vi "CODMn通讯.vi"() -> ()   [LabVIEW 2016, in "斯坦道CODMn.lvlib"]
uses:
  <vilib>/NI/Modbus Library/API/Wrapper/Create TCP Slave.vi
  <vilib>/NI/Modbus Library/API/slave/Modbus Slave.lvclass
  <vilib>/Plasmionique/MB Master/MB_Master/MB_Master.lvclass
  <vilib>/Plasmionique/MB Master/MB Master.lvlib
  <vilib>/Utility/config.llb/NI_LVConfig.lvlib
  <vilib>/NI/Modbus Library/API/Wrapper/API Main.lvlib
panel:
  in  "读取数据":bool
  in  "释放串口":bool
  in  "打开串口":bool
  out "队列中元素数量":i32
  out "元素":cluster{"命令":string}[](array[cluster])
  out "待处理插入数量":i32
  out "读取公式":u16[](array[numeric])
  out "读取参数":u16[](array[numeric])
  out "数据存储":u16[](array[numeric])
  out "温度":bool[](array[boolean])
  out "M输出点":bool[](array[boolean])
  out "ORP、时间":u16[](array[numeric])
  out "测量状态":u16[](array[numeric])
  out "通讯状态":bool
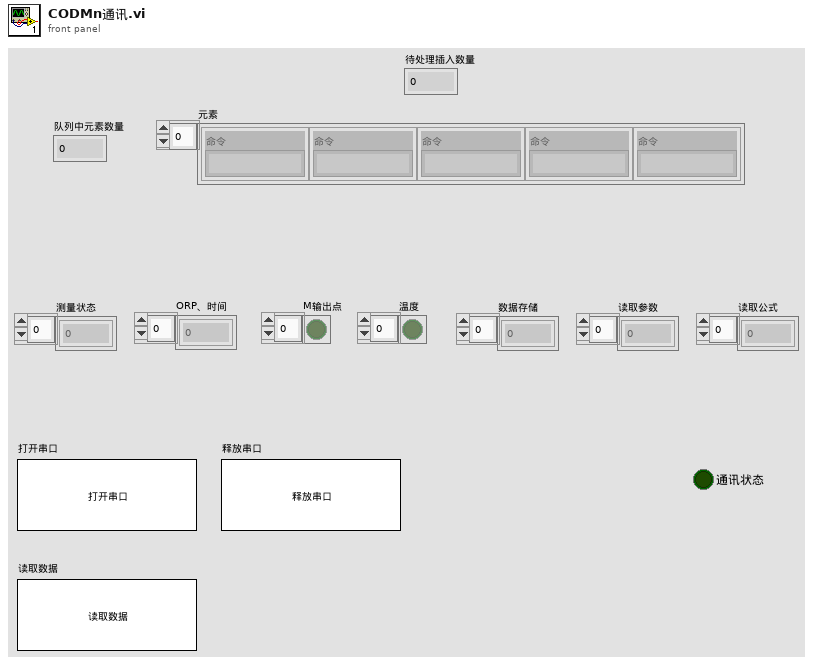
[diagram p1: front panel]
types:
  T1 = cluster{"命令":string, "测量模式":enum16{"水样测量", "标样核查", "零点核查", "跨度核查", "空白测试", "加标回收", "平行样", "校零", "校标"}, "CODMn量程切换":enum32{"H", "L", "AUTO"}}
  T2 = typedef "NI_LVConfig.lvlib/Config Data RefNum.ctl" = refnum<k1>
  T3 = enum16{"空闲", "水样测试", "标样核查", "零点核查", "跨度核查", "空白测试", "平行样测试", "质控样", "空白校准", "标样校准", "加标回收"}
  T4 = enum16{"水样测量", "标样核查", "零点核查", "跨度核查", "空白测试", "加标回收", "平行样", "校零", "校标"}
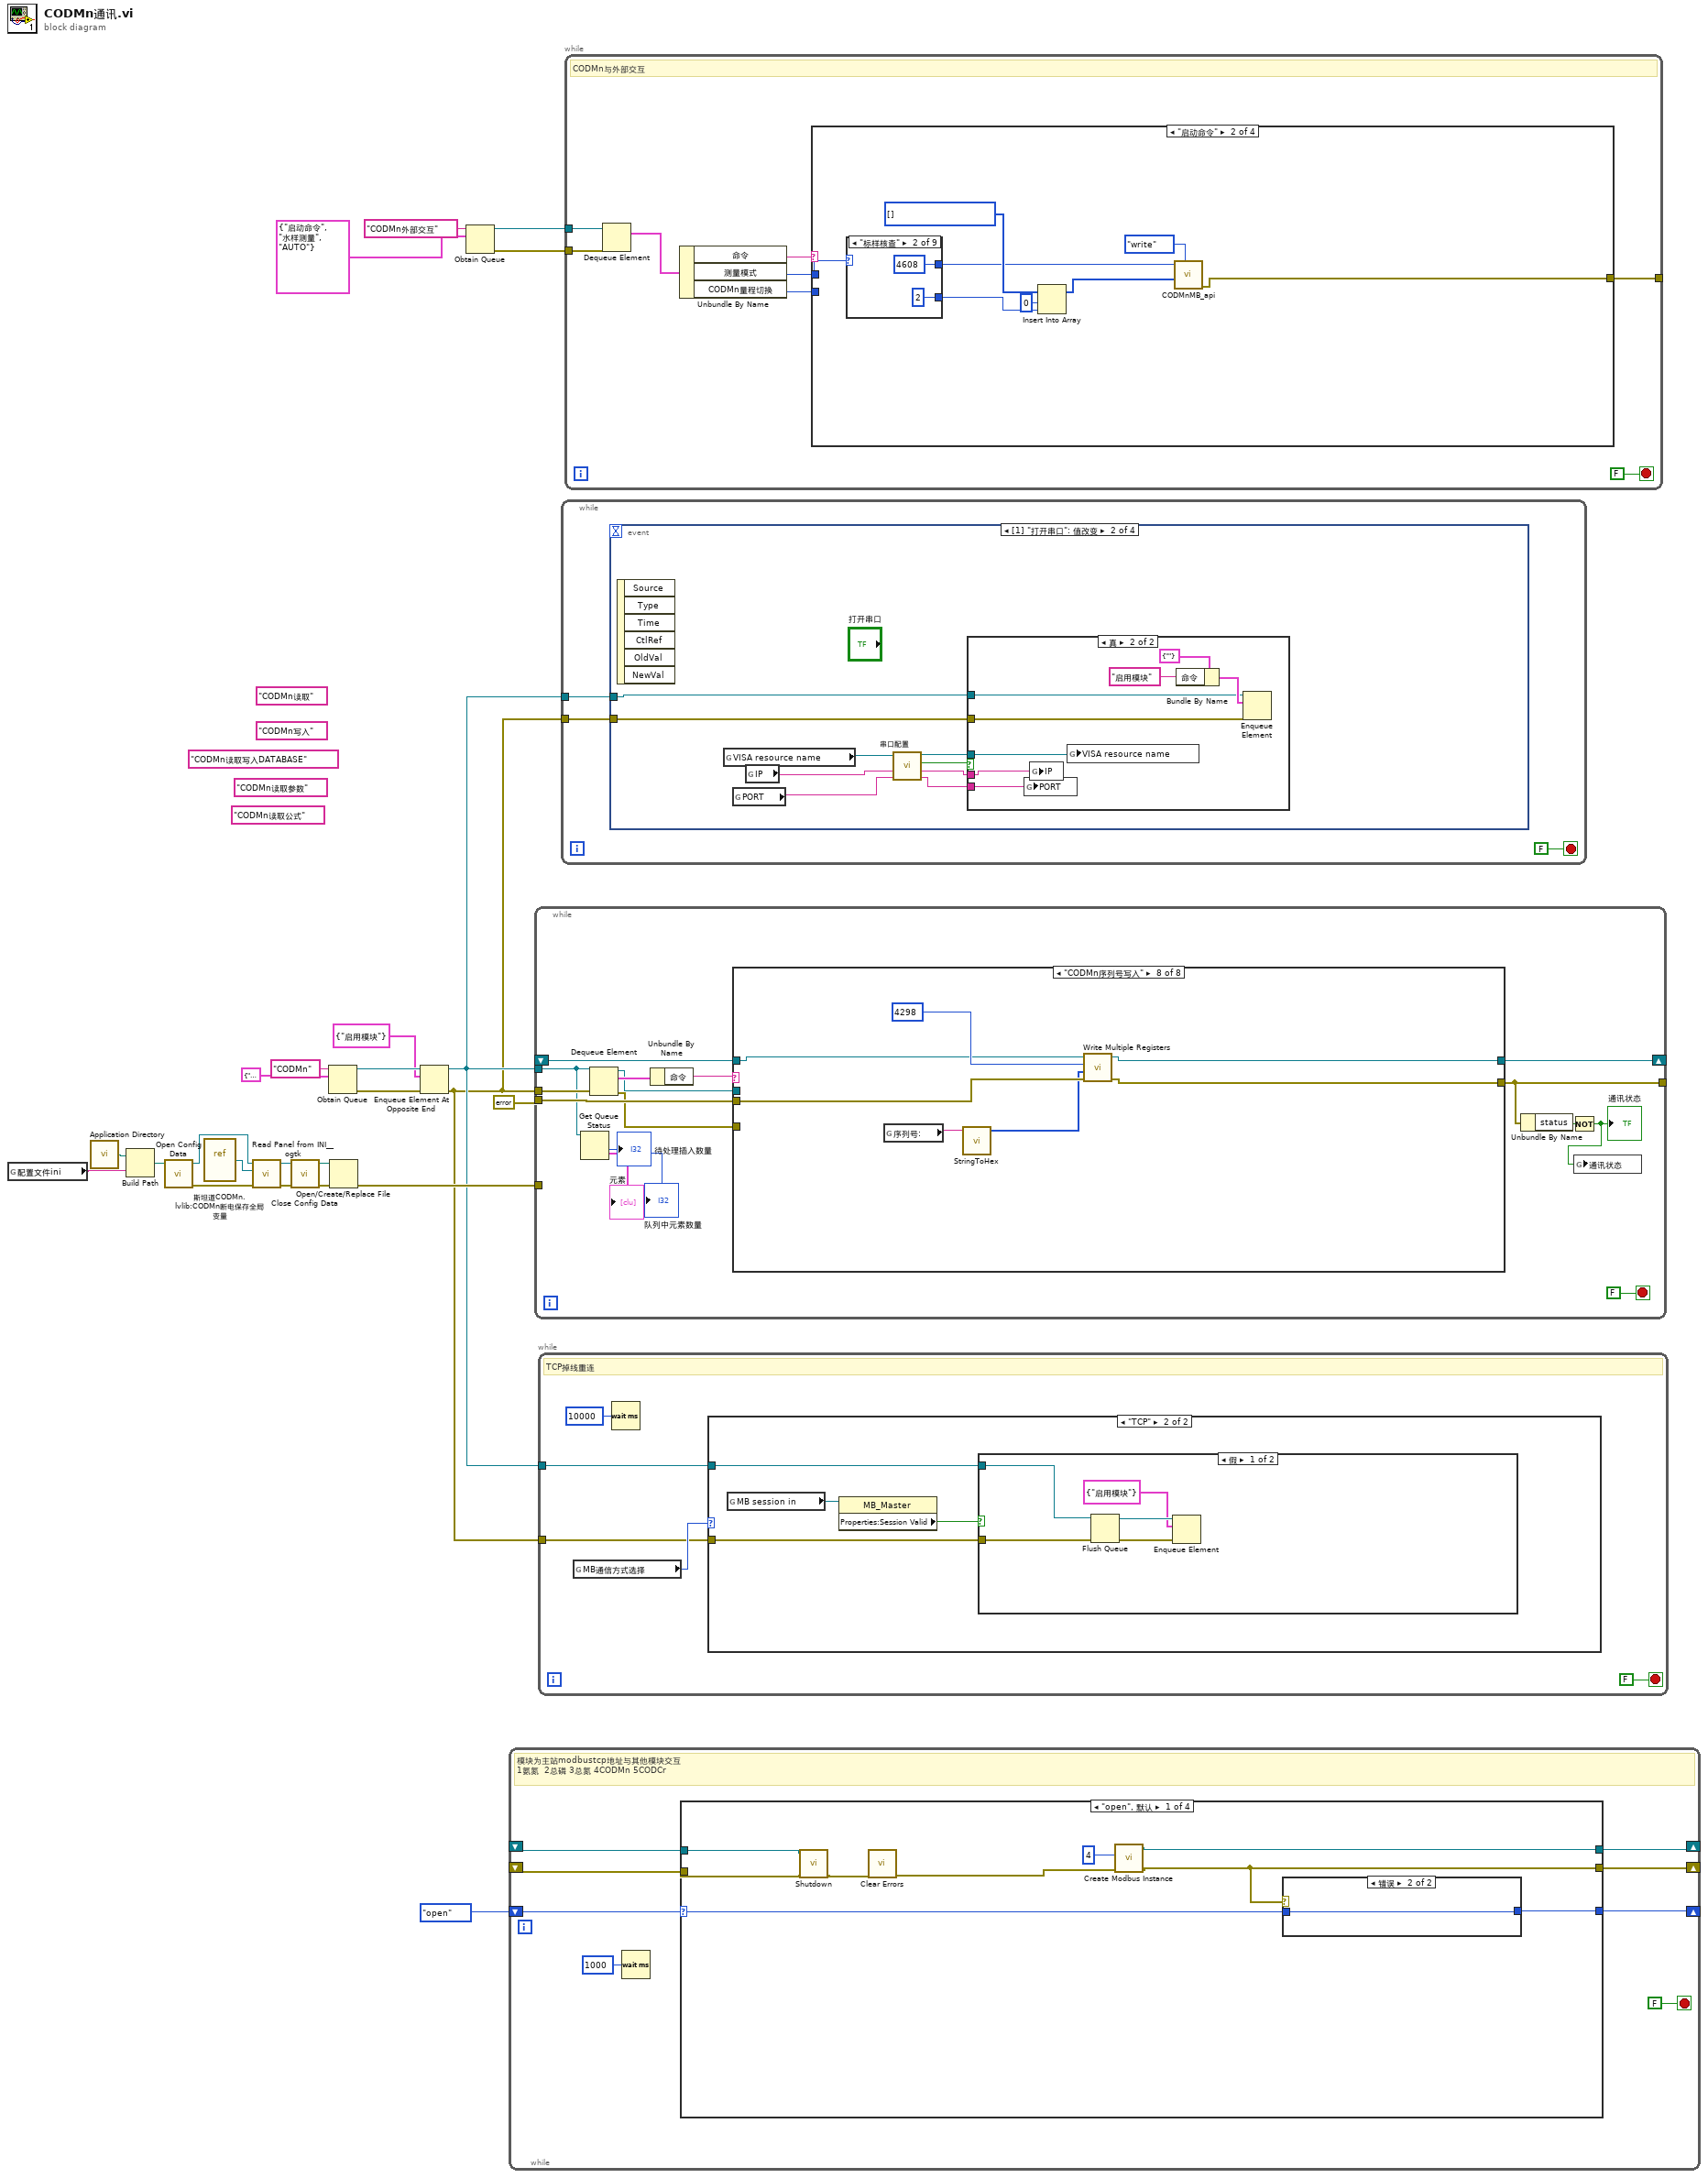
[diagram p0: block diagram]
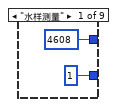
[diagram p3: hidden frame]
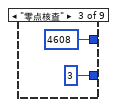
[diagram p4: hidden frame]
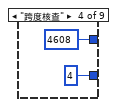
[diagram p5: hidden frame]
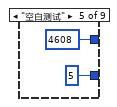
[diagram p6: hidden frame]
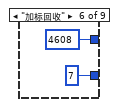
[diagram p7: hidden frame]
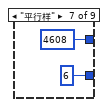
[diagram p8: hidden frame]
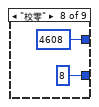
[diagram p9: hidden frame]
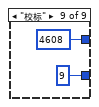
[diagram p10: hidden frame]
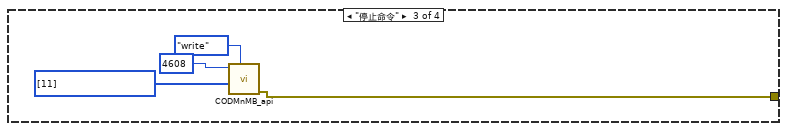
[diagram p11: hidden frame]
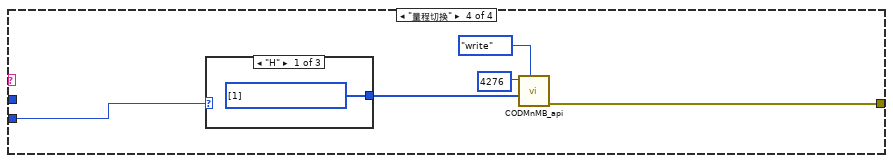
[diagram p12: hidden frame]
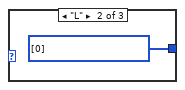
[diagram p13: hidden frame]
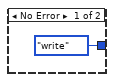
[diagram p17: hidden frame]
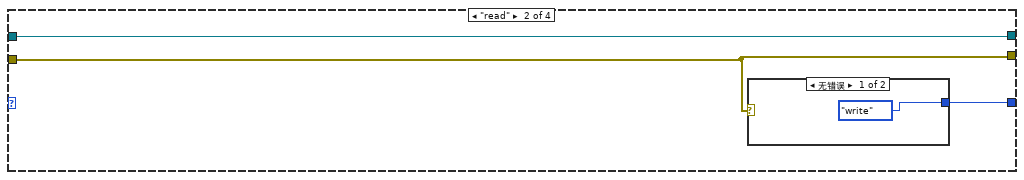
[diagram p18: hidden frame]
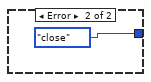
[diagram p19: hidden frame]
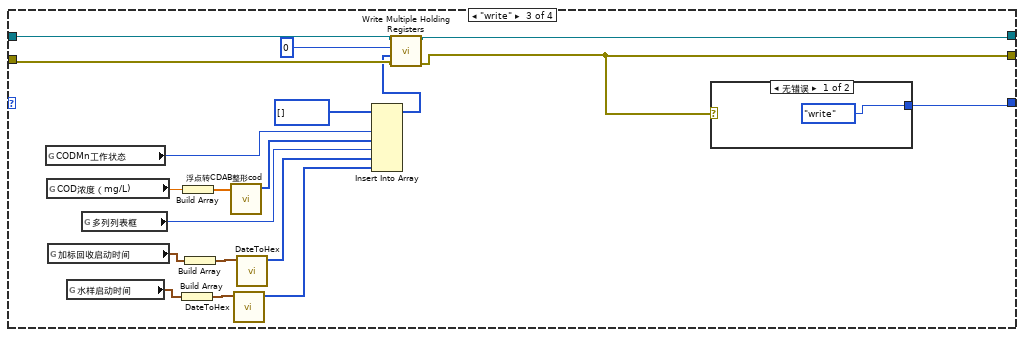
[diagram p20: hidden frame]
diagram:
  (unwired) "CODMn读取公式" ("名称（未命名）")
  (unwired) "CODMn读取写入DATABASE" ("名称（未命名）")
  (unwired) "CODMn读取参数" ("名称（未命名）")
  (unwired) "CODMn读取" ("名称（未命名）")
  (unwired) "CODMn写入" ("名称（未命名）")
  n1 = global read "COD内部交互全局.vi" "配置文件ini"() -> (w5:string)
  n2 = call <vilib>:"Application Directory.vi"() -> ("Application Directory"=w18:path)
  n3 = Build Path(base path=w18, name or relative path=w5) -> (appended path=w17:path)
  n4 = call <vilib>:"Open Config Data.vi"("configuration file path"=w17) -> ("error out"=w13:errorcluster, "refnum"=w16:T2)  [unwired: 8 in, 1 out]
  n5 = vi-ref "斯坦道CODMn.lvlib:CODMn断电保存全局变量.vi"() -> (w15:refnum<vi>)
  n6 = call <userlib>:"Read Panel from INI__ogtk.vi"("error in (no error)"=w13, "VI ref"=w15, "refnum"=w16) -> ("error out"=w12:errorcluster, "refnum out"=w14:T2)  [unwired: 7 in]
  n7 = call <vilib>:"Close Config Data.vi"("error in (no error)"=w12, "refnum"=w14) -> ("error out"=w11:errorcluster, "file path"=w10:path)  [unwired: 8 in]
  n8 = Obtain Queue(name (unnamed)="CODMn" ("名称（未命名）"), element data type=cluster{"命令":string} {"命令"="启用模块"} ("元素")) -> (queue out=w21:refnum<queue>, error out=w20:errorcluster)  [unwired: 3 in, 1 out]
  n9 = Open/Create/Replace File(file path (use dialog)=w10, error in=w11) -> (error out=w9:errorcluster)  [unwired: 4 in, 2 out]
  n10 = Enqueue Element At Opposite End(queue=w21, element=cluster{"命令":string} {"命令"="启用模块"} ("元素"), error in (no error)=w20) -> (queue out=w7:refnum<queue>, error out=w6:errorcluster)  [unwired: 1 in, 1 out]
  n11 = Obtain Queue(name (unnamed)="CODMn外部交互" ("名称（未命名）"), element data type=T1 {"命令"="启动命令", "测量模式"=enum."水样测量", "CODMn量程切换"=enum."AUTO"} ("元素")) -> (queue out=w2:refnum<queue>, error out=w1:errorcluster)  [unwired: 3 in, 1 out]
  n12 = while {
    shift-right: [w30] -> _
    shift-left: _ -> [w32]
    shift-right: [w29] -> _
    shift-left: _ -> [w31]
    shift-right: [w26] -> _
    shift-left: enum16{"open", "read", "write", "close"}."open" -> [w27]
    stop <- FALSE stop-if-true
    # "模块为主站modbustcp地址与其他模块交互\n1氨氮  2总磷 3总氮 4CODMn 5CODCr"
    n13 = Wait (ms)(milliseconds to wait=u32 1000 ("等待时间（毫秒）")) -> ()  [unwired: 1 out]
    n14 = case shown="\"open\", 默认" w27 {
      selector: w27 -> [w41 _ _ _]
      tunnel: w32 -> [w35 w44 w66 w72]
      tunnel: w31 -> [w34 w45 w63 w71]
      tunnel: [w38 w44 w65 w72] -> w30
      tunnel: [w37 w45 w64 w74] -> w29
      tunnel: [w40 w46 w67 enum16{"open", "read", "write", "close"}."open"] -> w26
      frame "open", Default {
        n15 = call-dynamic "Shutdown.vi"("error in"=w34, "Modbus slave in"=w35) -> ("error out"=w33:errorcluster)  [unwired: 9 in]
        n16 = call <vilib>:"Clear Errors.vi"("error in (no error)"=w33) -> ("error out"=w36:errorcluster)  [unwired: 5 in, 1 out]
        n17 = call-poly <vilib>:"Create Modbus Instance.vi"("error in"=w36, "port (502)"=u16 4) -> ("error out"=w37:errorcluster, "TCP slave instance"=w38:refnum<class "Modbus Slave.lvclass">)  [unwired: 8 in]
        n18 = case shown="错误" w37 {
          tunnel: w41 -> [_ w43]
          tunnel: [enum16{"open", "read", "write", "close"}."write" w43] -> w40
          frame No Error {
          }
          frame Error {
          }
        }
      }
      frame "read" {
        n19 = case shown="无错误" w45 {
          tunnel: [enum16{"open", "read", "write", "close"}."write" enum16{"open", "read", "write", "close"}."close"] -> w46
          frame No Error {
          }
          frame Error {
          }
        }
      }
      frame "write" {
        n20 = global read "COD测量模式全局.vi" "CODMn工作状态"() -> (w53:T3)
        n21 = global read "COD浓度全局变量.vi" "COD浓度（mg/L)"() -> (w55:dbl)
        n22 = global read "COD测量模式全局.vi" "加标回收启动时间"() -> (w58:timestamp)
        n23 = global read "COD测量模式全局.vi" "水样启动时间"() -> (w60:timestamp)
        n24 = global read "运行时序全局变量.vi" "多列列表框"() -> (w57:i32)
        n25 = Build Array(w60) -> (w59:timestamp[])
        n26 = Build Array(w55) -> (w54:dbl[])
        n27 = Build Array(w58) -> (w51:timestamp[])
        n28 = call "浮点转CDAB整形cod.vi"("浮点数"=w54) -> ("CDAB整形输出"=w56:u16[])  [unwired: 10 in]
        n29 = call "DateToHex.vi"("DATE"=w59) -> ("数组"=w62:u16[])  [unwired: 10 in]
        n30 = call "DateToHex.vi"("DATE"=w51) -> ("数组"=w61:u16[])  [unwired: 10 in]
        n31 = Insert Into Array(array=u16[] [] ("values"), new element #1=w53, new element #2=w56, new element #3=w57, new element #4=w61, new element #5=w62) -> (w50:u16[])  [unwired: 1 in]
        n32 = call-dynamic "Write Multiple Holding Registers.vi"("error in"=w63, "registers to write"=w50, "starting address"=u16 0, "Modbus slave in"=w66) -> ("error out"=w64:errorcluster, "Modbus slave out"=w65:refnum<class "Modbus Slave.lvclass">)  [unwired: 6 in]
        n33 = case shown="无错误" w64 {
          tunnel: [enum16{"open", "read", "write", "close"}."write" enum16{"open", "read", "write", "close"}."close"] -> w67
          frame No Error {
          }
          frame Error {
          }
        }
      }
      frame "close" {
        n34 = call-dynamic "Shutdown.vi"("error in"=w71, "Modbus slave in"=w72) -> ("error out"=w70:errorcluster)  [unwired: 9 in]
        n35 = call <vilib>:"Clear Errors.vi"("error in (no error)"=w70) -> ("error out"=w74:errorcluster)  [unwired: 5 in, 1 out]
      }
    }
  }
  n36 = while {
    tunnel: w7 -> [w80]
    tunnel: w6 -> [w89]
    tunnel: [w81] -> _
    shift-right: [w85] -> _
    shift-left: _ -> [w84]
    tunnel: errorcluster {"status"=FALSE, "code"=0, "source"=""} ("error out") -> [w83]
    tunnel: w9 -> [_]
    stop <- FALSE stop-if-true
    n37 = Get Queue Status(queue=w80) -> (# pending insert=→"待处理插入数量":i32, # elements in queue=→"队列中元素数量":i32, elements=→"元素":cluster{"命令":string}[])  [unwired: 2 in, 5 out]
    n38 = Dequeue Element(queue=w80, error in (no error)=w89) -> (queue out=w76:refnum<queue>, element=w88:cluster{"命令":string}, error out=w75:errorcluster)  [unwired: 1 in, 1 out]
    n39 = Unbundle By Name(w88) -> ("命令"=w87:string)
    n40 = case shown="\"CODMn序列号写入\"" w87 {
      tunnel: [w92 w96 w107 w118 w139 w148 w165 w172] -> w85
      tunnel: [w91 w93 w108 w111 w137 w147 w164 w171] -> w81
      tunnel: w84 -> [w92 _ _ w132 w143 w157 w168 w176]
      tunnel: w83 -> [w91 w97 w109 w131 w140 w156 w167 w175]
      tunnel: w76 -> [_ w95 _ _ _ _ _ _]
      tunnel: w75 -> [_ w94 _ _ _ _ _ _]
      frame Default {
      }
      frame "启用模块" {
        n41 = call "CODMnMB_api.vi"("STEP"=enum16{"open", "read", "write", "close"}."open", "Error in"=w97) -> ("error out"=w93:errorcluster, "MB session out"=w96:refnum<class "MB_Master.lvclass">)  [unwired: 7 in, 1 out]
        n42 = case shown="无错误" w93 {
          tunnel: w95 -> [w103 _]
          tunnel: w94 -> [w100 _]
          frame No Error {
            n43 = global read "COD内部交互全局.vi" "序列号:"() -> (w102:string)
            n44 = Empty String/Path?(string/path=w102) -> (empty?=w101:bool)
            n45 = Not(x=w101) -> (.not. x?=w99:bool)
            n46 = case shown="真" w99 {
              tunnel: w103 -> [_ w106]
              tunnel: w100 -> [_ w105]
              frame False {
              }
              frame True {
                # "发货调试版用"
                n47 = Enqueue Element(queue=w106, element=cluster{"命令":string} {"命令"="CODMn序列号写入"} ("元素"), error in (no error)=w105) -> ()  [unwired: 1 in, 3 out]
              }
            }
          }
          frame Error {
          }
        }
        n48 = global write "COD浓度全局变量.vi" "MB session in"(w96) -> ()
      }
      frame "停用模块" {
        n49 = call "CODMnMB_api.vi"("STEP"=enum16{"open", "read", "write", "close"}."close", "Error in"=w109) -> ("error out"=w108:errorcluster, "MB session out"=w107:refnum<class "MB_Master.lvclass">)  [unwired: 7 in, 1 out]
      }
      frame "CODMn读取" {
        n50 = call <vilib>:"Read Holding Registers.vi"("error in (no error)"=w131, "quantity"=u16 50 ("number of holding registers"), "starting address"=u16 4224, "MB session in"=w132) -> ("error out"=w122:errorcluster, "Registers"=w128:u16[], "MB session out"=w123:refnum<class "MB_Master.lvclass">)  [unwired: 5 in]
        n51 = case shown="无错误" w122 {
          tunnel: w128 -> [w136 _]
          frame No Error {
            n52 = global write "COD内部交互全局.vi" "测量状态"(w136) -> ()
            "测量状态" <- w136
          }
          frame Error {
          }
        }
        n53 = call <vilib>:"Read Holding Registers.vi"("error in (no error)"=w122, "quantity"=u16 10, "starting address"=u16 4101, "MB session in"=w123) -> ("error out"=w117:errorcluster, "Registers"=w121:u16[], "MB session out"=w120:refnum<class "MB_Master.lvclass">)  [unwired: 5 in]
        n54 = case shown="无错误" w117 {
          tunnel: w121 -> [w135 _]
          frame No Error {
            n55 = global write "COD内部交互全局.vi" "ORP、时间"(w135) -> ()
            "ORP、时间" <- w135
          }
          frame Error {
          }
        }
        n56 = call <vilib>:"Read Coils.vi"("error in (no error)"=w117, "quantity"=u16 11, "starting address"=u16 137, "MB session in"=w120) -> ("error out"=w115:errorcluster, "Coils"=w116:bool[], "MB session out"=w119:refnum<class "MB_Master.lvclass">)  [unwired: 5 in]
        n57 = case shown="无错误" w115 {
          tunnel: w116 -> [w134 _]
          frame No Error {
            n58 = global write "COD内部交互全局.vi" "M输出点"(w134) -> ()
            "M输出点" <- w134
          }
          frame Error {
          }
        }
        n59 = call <vilib>:"Read Coils.vi"("error in (no error)"=w115, "quantity"=u16 1, "starting address"=u16 400, "MB session in"=w119) -> ("error out"=w111:errorcluster, "Coils"=w112:bool[], "MB session out"=w118:refnum<class "MB_Master.lvclass">)  [unwired: 5 in]
        n60 = case shown="无错误" w111 {
          tunnel: w112 -> [w133 _]
          frame No Error {
            n61 = global write "COD内部交互全局.vi" "温度"(w133) -> ()
            "温度" <- w133
          }
          frame Error {
          }
        }
      }
      frame "CODMn读取写入DATABASE" {
        n62 = call <vilib>:"Read Holding Registers.vi"("error in (no error)"=w140, "quantity"=u16 10 ("number of holding registers"), "starting address"=u16 4101, "MB session in"=w143) -> ("error out"=w137:errorcluster, "Registers"=w138:u16[], "MB session out"=w139:refnum<class "MB_Master.lvclass">)  [unwired: 5 in]
        n63 = case shown="无错误" w137 {
          tunnel: w138 -> [w145 _]
          frame No Error {
            n64 = global write "COD内部交互全局.vi" "数据存储"(w145) -> ()
            n65 = global write "COD内部交互全局.vi" "读取写入data"(TRUE ("读取参数显示")) -> ()
            "数据存储" <- w145
          }
          frame Error {
          }
        }
      }
      frame "CODMn读取参数" {
        n66 = call <vilib>:"Read Holding Registers.vi"("error in (no error)"=w156, "quantity"=u16 35 ("number of holding registers"), "starting address"=u16 4272, "MB session in"=w157) -> ("error out"=w151:errorcluster, "Registers"=w153:u16[], "MB session out"=w152:refnum<class "MB_Master.lvclass">)  [unwired: 5 in]
        n67 = case shown="无错误" w151 {
          tunnel: w153 -> [w161 _]
          frame No Error {
            n68 = global write "COD内部交互全局.vi" "读取参数"(w161) -> ()
            n69 = global write "COD内部交互全局.vi" "读取参数显示"(TRUE ("读取参数显示")) -> ()
            "读取参数" <- w161
          }
          frame Error {
          }
        }
        n70 = call <vilib>:"Read Holding Registers.vi"("error in (no error)"=w151, "quantity"=u16 4, "starting address"=u16 5596, "MB session in"=w152) -> ("error out"=w147:errorcluster, "Registers"=w146:u16[], "MB session out"=w148:refnum<class "MB_Master.lvclass">)  [unwired: 5 in]
        n71 = case shown="无错误" w147 {
          tunnel: w146 -> [w159 _]
          frame No Error {
            n72 = global write "COD内部交互全局.vi" "读取浮台参数"(w159) -> ()
            n73 = global write "COD内部交互全局.vi" "读取浮台参数显示"(TRUE ("读取参数显示")) -> ()
          }
          frame Error {
          }
        }
      }
      frame "CODMn读取公式" {
        n74 = call <vilib>:"Read Holding Registers.vi"("error in (no error)"=w167, "quantity"=u16 94 ("number of holding registers"), "starting address"=u16 4616, "MB session in"=w168) -> ("error out"=w164:errorcluster, "Registers"=w166:u16[], "MB session out"=w165:refnum<class "MB_Master.lvclass">)  [unwired: 5 in]
        n75 = case shown="无错误" w164 {
          tunnel: w166 -> [w170 _]
          frame No Error {
            n76 = global write "COD内部交互全局.vi" "读取公式"(w170) -> ()
            n77 = global write "COD内部交互全局.vi" "读取公式显示"(TRUE ("读取参数显示")) -> ()
            "读取公式" <- w170
          }
          frame Error {
          }
        }
      }
      frame "CODMn序列号写入" {
        n78 = global read "COD内部交互全局.vi" "序列号:"() -> (w174:string)
        n79 = call "StringToHex.vi"("STRING"=w174) -> ("数组"=w173:u16[])  [unwired: 10 in]
        n80 = call <vilib>:"Write Multiple Registers.vi"("error in (no error)"=w175, "values"=w173, "starting address"=u16 4298, "MB session in"=w176) -> ("error out"=w171:errorcluster, "MB session out"=w172:refnum<class "MB_Master.lvclass">)  [unwired: 6 in]
      }
    }
    n81 = Unbundle By Name(w81) -> ("status"=w86:bool)
    n82 = Not(x=w86) -> (.not. x?=w82:bool)
    "通讯状态" <- w82
    n83 = global write "COD内部交互全局.vi" "通讯状态"(w82) -> ()
  }
  n84 = while "While循环" {
    tunnel: w7 -> [w179]
    tunnel: w6 -> [w178]
    stop <- FALSE stop-if-true
    # "TCP掉线重连"
    n85 = global read "CODMn断电保存全局变量.vi" "MB通信方式选择"() -> (w180:enum16{"串口", "TCP"})
    n86 = Wait (ms)(milliseconds to wait=u32 10000 ("等待时间（毫秒）")) -> ()  [unwired: 1 out]
    n87 = case shown="\"TCP\"" w180 {
      tunnel: w179 -> [_ w184]
      tunnel: w178 -> [_ w183]
      frame "串口", Default {
      }
      frame "TCP" {
        n88 = global read "COD浓度全局变量.vi" "MB session in"() -> (w186:refnum<class "MB_Master.lvclass">)
        n89 = property class="MB_Master"(reference=w186) -> ("Properties:Session Valid"=w185:bool)  [unwired: 1 in, 2 out]
        n90 = case shown="假" w185 {
          tunnel: w184 -> [w188 _]
          tunnel: w183 -> [w187 _]
          frame False {
            n91 = Flush Queue(queue=w188, error in (no error)=w187) -> (queue out=w191:refnum<queue>, error out=w190:errorcluster)  [unwired: 1 out]
            n92 = Enqueue Element(queue=w191, element=cluster{"命令":string} {"命令"="启用模块"} ("元素"), error in (no error)=w190) -> ()  [unwired: 1 in, 3 out]
          }
          frame True {
          }
        }
      }
    }
  }
  n93 = while {
    tunnel: w7 -> [w193]
    tunnel: w6 -> [w192]
    stop <- FALSE stop-if-true
    n94 = event shown="[1] \"打开串口\": 值改变" {
      selector: _ -> [_ _ _ _]
      dyn-events: _ -> [_ _ _ _]
      timeout: _ -> [_ _ _ _]
      tunnel: w193 -> [_ w200 w214 w216]
      tunnel: w192 -> [_ w199 w213 w215]
      event Timeout {
        n95 = event-data() -> ()  [unwired: 1 in, 3 out]
      }
      event "打开串口": Value Change {
        n96 = event-data() -> ()  [unwired: 1 in, 6 out]
        n97 = global read "CODMn断电保存全局变量.vi" "VISA resource name"() -> (w203:refnum<visa-resource-name>)
        n98 = global read "CODMn断电保存全局变量.vi" "PORT"() -> (w195:string)
        n99 = global read "CODMn断电保存全局变量.vi" "IP"() -> (w196:string)
        n100 = call "串口配置.vi"("PORT"=w195, "IP"=w196, "请选择串口:"=w203) -> ("PORT 2"=w197:string, "IP 2"=w198:string, "确认 2"=w201:bool, "VISA资源名称 2"=w202:refnum<visa-resource-name>)  [unwired: 4 in, 1 out]
        n101 = case shown="真" w201 {
          tunnel: w202 -> [_ w211]
          tunnel: w200 -> [_ w207]
          tunnel: w199 -> [_ w206]
          tunnel: w198 -> [_ w205]
          tunnel: w197 -> [_ w204]
          frame False {
          }
          frame True {
            n102 = global write "CODMn断电保存全局变量.vi" "PORT"(w204) -> ()
            n103 = global write "CODMn断电保存全局变量.vi" "IP"(w205) -> ()
            n104 = global write "CODMn断电保存全局变量.vi" "VISA resource name"(w211) -> ()
            n105 = Bundle By Name(cluster=cluster{"命令":string} {"命令"=""} ("元素"), "命令"="启用模块" ("名称（未命名）")) -> (w208:cluster{"命令":string})
            n106 = Enqueue Element(queue=w207, element=w208, error in (no error)=w206) -> ()  [unwired: 1 in, 3 out]
          }
        }
      }
      event "释放串口": Value Change {
        n107 = event-data() -> ()  [unwired: 1 in, 6 out]
        n108 = Enqueue Element(queue=w214, element=cluster{"命令":string} {"命令"="停用模块"} ("元素"), error in (no error)=w213) -> ()  [unwired: 1 in, 3 out]
      }
      event "读取数据": Value Change {
        n109 = event-data() -> ()  [unwired: 1 in, 6 out]
        n110 = Enqueue Element(queue=w216, element=cluster{"命令":string} {"命令"="CODMn读取"} ("元素"), error in (no error)=w215) -> ()  [unwired: 1 in, 3 out]
      }
    }
  }
  n111 = while {
    tunnel: w2 -> [w223]
    tunnel: w1 -> [w222]
    tunnel: [w218] -> _
    stop <- FALSE stop-if-true
    # "CODMn与外部交互"
    n112 = Dequeue Element(queue=w223, error in (no error)=w222) -> (element=w224:T1)  [unwired: 1 in, 3 out]
    n113 = Unbundle By Name(w224) -> ("命令"=w221:string, "测量模式"=w220:T4, "CODMn量程切换"=w219:enum32{"H", "L", "AUTO"})
    n114 = case shown="\"启动命令\"" w221 {
      tunnel: w220 -> [_ w227 _ _]
      tunnel: w219 -> [_ _ _ w257]
      tunnel: [_ w226 w252 w256] -> w218
      frame "假", Default {
      }
      frame "启动命令" {
        n115 = case shown="\"标样核查\"" w227 {
          tunnel: [u16 4608 ("address") u16 4608 ("address") u16 4608 ("address") u16 4608 ("address") u16 4608 ("address") u16 4608 ("address") u16 4608 ("address") u16 4608 ("address") u16 4608 ("address")] -> w229
          tunnel: [u16 1 ("address") u16 2 ("address") u16 3 ("address") u16 4 ("address") u16 5 ("address") u16 7 ("address") u16 6 ("address") u16 8 ("address") u16 9 ("address")] -> w233
          frame "水样测量" {
          }
          frame "标样核查" {
          }
          frame "零点核查" {
          }
          frame "跨度核查" {
          }
          frame "空白测试" {
          }
          frame "加标回收" {
          }
          frame "平行样" {
          }
          frame "校零" {
          }
          frame "校标" {
          }
        }
        n116 = Insert Into Array(array=u16[] [] ("values"), index=0 ("索引"), new element=w233) -> (w228:u16[])
        n117 = call "CODMnMB_api.vi"("STEP"=enum16{"open", "read", "write", "close"}."write", "values"=w228, "starting address"=w229) -> ("error out"=w226:errorcluster)  [unwired: 6 in, 2 out]
      }
      frame "停止命令" {
        n118 = call "CODMnMB_api.vi"("STEP"=enum16{"open", "read", "write", "close"}."write", "values"=u16[] [11], "starting address"=u16 4608) -> ("error out"=w252:errorcluster)  [unwired: 6 in, 2 out]
      }
      frame "量程切换" {
        n119 = case shown="\"H\"" w257 {
          tunnel: [u16[] [1] ("values") u16[] [0] ("values") _] -> w260
          frame "H" {
          }
          frame "L" {
          }
          frame "AUTO", Default {
          }
        }
        n120 = call "CODMnMB_api.vi"("STEP"=enum16{"open", "read", "write", "close"}."write", "values"=w260, "starting address"=u16 4276) -> ("error out"=w256:errorcluster)  [unwired: 6 in, 2 out]
      }
    }
  }
